vi "Experiment-2-5-1.vi"() -> ()   [LabVIEW 2014]
panel:
  out "Closed-form series":dbl
  out "Absolute error":dbl
  out "Sum of geometric series":dbl
  in  "iteration":i32
  in  "Input x (-1 < x < 1)":dbl
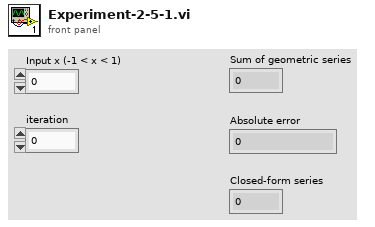
[diagram p1: front panel]
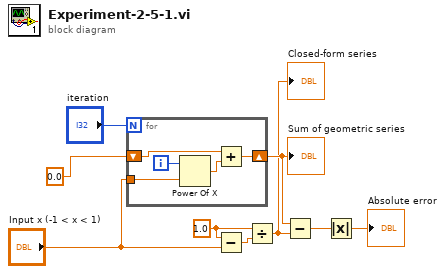
[diagram p0: block diagram]
diagram:
  w7 = 1.0
  n1 = for {
    N: "iteration" -> [_]
    tunnel: "Input x (-1 < x < 1)" -> [w13]
    shift-right: [w12] -> w3
    shift-left: 0.0 -> [w11]
    i -> [w14]
    n2 = Power Of X(1:w13, 2:w14) -> (0:w10:dbl)
    n3 = Add(x=w11, y=w10) -> (x+y=w12:dbl)
  }
  "Sum of geometric series" <- w3
  n4 = Subtract(x=w7, y="Input x (-1 < x < 1)") -> (x-y=w6:dbl)
  n5 = Divide(x=w7, y=w6) -> (x/y=w2:dbl)
  "Closed-form series" <- w2
  n6 = Subtract(x=w3, y=w2) -> (x-y=w4:dbl)
  n7 = Absolute Value(x=w4) -> (abs(x)=→"Absolute error":dbl)
